vi "FitParametersPixel2RAW.vi"(9 "Subsampling":u16=1, 10 "ROI Offset":i32[](array[numeric]), 11 "Fits Pixel":dbl[](array[numeric])) -> (3 "Fit RAW":dbl[](array[numeric]))   [LabVIEW 2015]
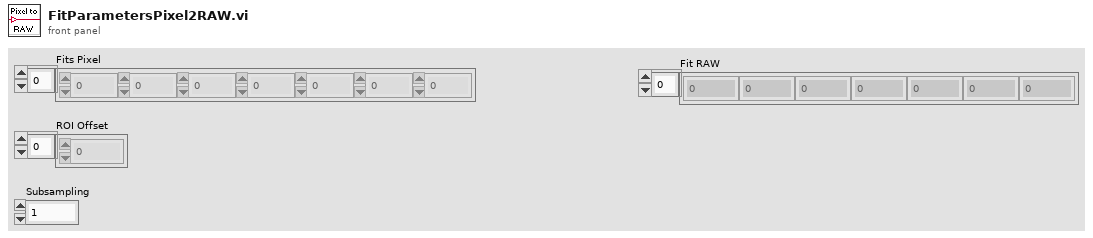
[diagram p1: front panel]
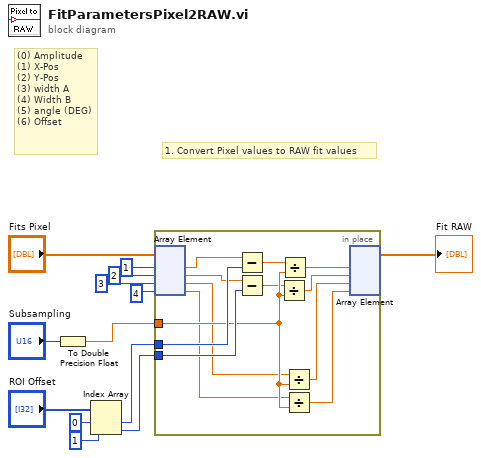
[diagram p0: block diagram]
diagram:
  # "1. Convert Pixel values to RAW fit values"
  # "(0) Amplitude\n(1) X-Pos\n(2) Y-Pos\n(3) width A\n(4) Width B\n(5) angle (DEG)\n(6) Offset"
  n1 = To Double Precision Float(number="Subsampling") -> (double precision float=w1:dbl)
  n2 = Index Array(array="ROI Offset", index #1=0 ("index"), index #2=1 ("index")) -> (element #1=w3:i32, element #2=w2:i32)
  n3 = in-place {
    in-place-border: w1 -> [w24]
    in-place-border: w3 -> [w26]
    in-place-border: w2 -> [w25]
    n4 = in-place-array #1("Fits Pixel", 1 ("index"), 2 ("index"), 3 ("index"), 4 ("index")) -> (w19:dbl, w18:dbl, w23:dbl, w22:dbl)
    n5 = Subtract(x=w19, y=w26) -> (x-y=w16:dbl)
    n6 = Subtract(x=w18, y=w25) -> (x-y=w14:dbl)
    n7 = Divide(x=w14, y=w24) -> (x/y=w15:dbl)
    n8 = Divide(x=w16, y=w24) -> (x/y=w17:dbl)
    n9 = Divide(x=w23, y=w24) -> (x/y=w21:dbl)
    n10 = Divide(x=w22, y=w24) -> (x/y=w20:dbl)
    n11 = in-place-array #1(w17, w15, w21, w20) -> (→"Fit RAW":dbl[])  [unwired: 4 out]
  }
